vi "Actor Core.vi"(8 "error in":errorcluster, 11 "Nested in":refnum<class "UI VISA Terminal.lvclass">) -> (0 "error out":errorcluster, 3 "Actor out":refnum<class "Actor.lvclass">)   [LabVIEW 2025, in "UI VISA Terminal.lvlib" / "UI VISA Terminal.lvclass"]
doc: "(<B>Filename</B>: Actor Framework.lvlib:Actor.lvclass:Actor Core.vi)\n\nReceives messages to the actor, reacts to them, and initiates any error handling that may shut the actor down.\n\nDescendant classes may override this VI to append parallel tasks for the actor to complete while it handles messages. Overrides use the Call Parent Method node."
uses:
  UI VISA Terminal.lvclass
  <vilib>/ActorFramework/Actor/Actor.lvclass
  UI VISA Terminal.lvclass/UI VISA Terminal.ctl
  <vilib>/ActorFramework/Actor/Actor.lvclass/Actor.ctl
  <vilib>/ActorFramework/Message Enqueuer/Message Enqueuer.lvclass/Message Enqueuer.ctl
  UI VISA Terminal Messages/Write Command Msg/Write Command Msg.lvclass/Write Command Msg.ctl
  UI VISA Terminal Messages/Open Session Msg/Open Session Msg.lvclass/Open Session Msg.ctl
  <vilib>/ActorFramework/Message Enqueuer/Init from Existing Queue.vi
  <vilib>/ActorFramework/Message Enqueuer/Enqueue.vi
  <vilib>/ActorFramework/Stop Msg/Stop Msg.lvclass
  UI VISA Terminal Messages/Write Command Msg/Write Command Msg.lvclass
  UI VISA Terminal Messages/Open Session Msg/Open Session Msg.lvclass
  UI VISA Terminal Messages/Close Session Msg/Close Session Msg.lvclass
  UI VISA Terminal Messages/Write Msg/Write Msg.lvclass
  UI VISA Terminal Messages/Read Msg/Read Msg.lvclass
  UI VISA Terminal Messages/Query Msg/Query Msg.lvclass
  <vilib>/ActorFramework/Message Priority Queue/Priority Enqueue.vi
  <vilib>/ActorFramework/Message Enqueuer/Message Enqueuer.lvclass
panel:
  in  "Query":bool
  in  "Read":bool
  in  "Write":bool
  in  "VISA resource name":refnum<visa-resource-name>
  in  "Stop":bool
  in  "Start":bool
  in  "Command":string
  out "Reply":string
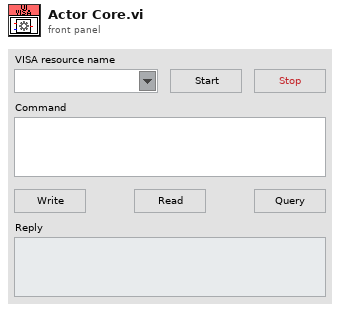
[diagram p1: front panel]
types:
  T1 = cluster{"Stop":refnum<user-event>, "Reply":refnum<user-event>}
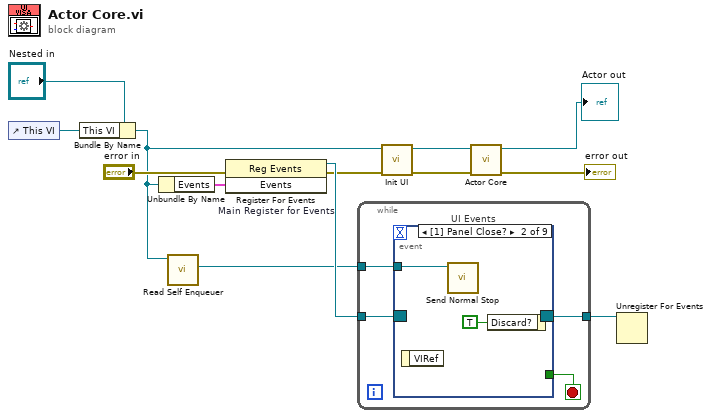
[diagram p0: block diagram]
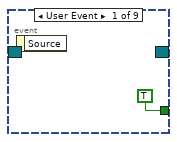
[diagram p2: hidden frame]
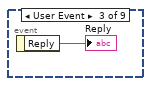
[diagram p3: hidden frame]
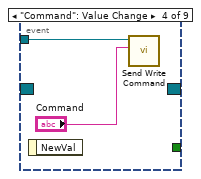
[diagram p4: hidden frame]
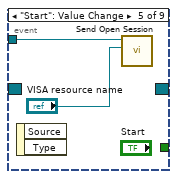
[diagram p5: hidden frame]
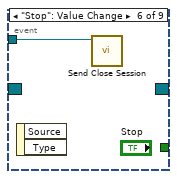
[diagram p6: hidden frame]
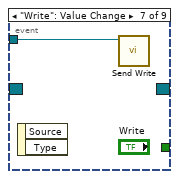
[diagram p7: hidden frame]
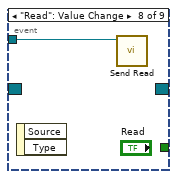
[diagram p8: hidden frame]
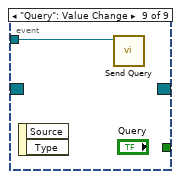
[diagram p9: hidden frame]
diagram:
  n1 = control-ref of="This VI"() -> (w5:refnum<vi>)
  n2 = Bundle By Name(cluster="Nested in", "This VI"=w5) -> (w2:refnum<class "UI VISA Terminal.lvclass">)
  n3 = Unbundle By Name(w2) -> ("Events"=w10:T1)
  n4 = call <vilib>:"Read Self Enqueuer.vi"("Actor"=w2) -> ("Self Enqueuer"=w8:refnum<class "Message Enqueuer.lvclass">)  [unwired: 10 in]
  n5 = register-events "Main Register for Events"(error in="error in", w10) -> (reference out=w11:refnum<event-registration>, error out=w6:errorcluster)  [unwired: 1 in]
  n6 = while {
    tunnel: w11 -> [w17]
    tunnel: [w15] -> w9
    tunnel: w8 -> [w14]
    stop <- w16 stop-if-true
    n7 = event "UI Events" shown="[1] Panel Close?" {
      selector: w17 -> [_ _ _ _ _ _ _ _ _]
      dyn-events: [_ _ _ _ _ _ _ _ _] -> w15
      timeout: _ -> [_ _ _ _ _ _ _ _ _]
      tunnel: [TRUE _ _ _ _ _ _ _ _] -> w16
      tunnel: w14 -> [_ w19 _ w23 w25 w26 w27 w28 w29]
      event User Event {
        n8 = event-data() -> ()  [unwired: 1 in, 1 out]
      }
      event Panel Close? {
        n9 = event-data() -> ()  [unwired: 1 in, 1 out]
        n10 = call <vilib>:"Send Normal Stop.vi"("Message Enqueuer"=w19) -> ()  [unwired: 10 in, 1 out]
        n11 = event-data("Discard?"=TRUE) -> ()  [unwired: 1 in, 1 out]
      }
      event User Event {
        n12 = event-data() -> ("Reply"=→"Reply":string)  [unwired: 1 in]
      }
      event "Command": Value Change {
        n13 = event-data() -> ()  [unwired: 1 in, 1 out]
        n14 = call "Send Write Command.vi"("Command"="Command", "Message Enqueuer"=w23) -> ()  [unwired: 8 in, 2 out]
      }
      event "Start": Value Change {
        n15 = event-data() -> ()  [unwired: 1 in, 2 out]
        n16 = call "Send Open Session.vi"("VISA resource name"="VISA resource name", "Message Enqueuer"=w25) -> ()  [unwired: 8 in, 2 out]
      }
      event "Stop": Value Change {
        n17 = event-data() -> ()  [unwired: 1 in, 2 out]
        n18 = call "Send Close Session.vi"("Message Enqueuer"=w26) -> ()  [unwired: 9 in, 2 out]
      }
      event "Write": Value Change {
        n19 = event-data() -> ()  [unwired: 1 in, 2 out]
        n20 = call "Send Write.vi"("Message Enqueuer"=w27) -> ()  [unwired: 9 in, 2 out]
      }
      event "Read": Value Change {
        n21 = event-data() -> ()  [unwired: 1 in, 2 out]
        n22 = call "Send Read.vi"("Message Enqueuer"=w28) -> ()  [unwired: 9 in, 2 out]
      }
      event "Query": Value Change {
        n23 = event-data() -> ()  [unwired: 1 in, 2 out]
        n24 = call "Send Query.vi"("Message Enqueuer"=w29) -> ()  [unwired: 9 in, 2 out]
      }
    }
  }
  n25 = call-dynamic "Init UI.vi"("error in (no error)"=w6, "UI VISA Terminal in"=w2) -> ("error out"=w3:errorcluster, "UI VISA Terminal out"=w1:refnum<class "UI VISA Terminal.lvclass">)  [unwired: 8 in]
  n26 = call-parent "Actor Core.vi"("error in"=w3, "Actor in"=w1) -> ("error out"=→"error out":errorcluster, "Actor out"=→"Actor out":refnum<class "Actor.lvclass">)  [unwired: 8 in]
  n27 = Unregister For Events(event registration refnum=w9) -> ()  [unwired: 1 in, 1 out]
